vi "File_Application Path Keeper.vi"(6 "Skip Dialogue":bool, 8 "Error":errorcluster, 11 "File Keeper Files":T1) -> (0 "Error Out":errorcluster, 2 "Valid Item Out":bool, 3 "Path Out":path=path "D:/Pitney PTS/PTS PROGRAMS/2-Sparks 1 and 2/SparksMain32.vi")   [LabVIEW 2015]
uses:
  TypeDefs_Utility/ENUM_File Keeper List.ctl
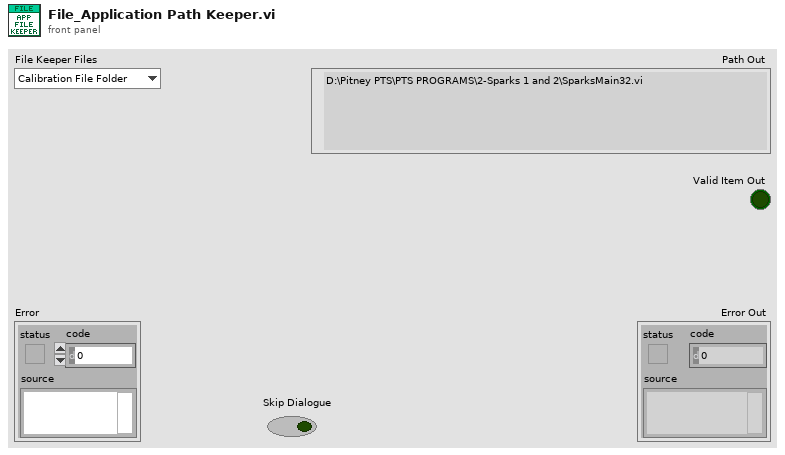
[diagram p1: front panel]
types:
  T1 = typedef "ENUM_File Keeper List.ctl" = enum16{"Calibration File Folder", "PNG Image Folder", "CSV File Folder"}
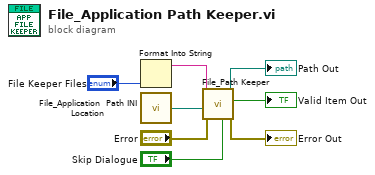
[diagram p0: block diagram]
diagram:
  n1 = Format Into String("File Keeper Files") -> (resulting string=w6:string)  [unwired: 3 in, 1 out]
  n2 = call "File_Application  Path INI Location.vi"() -> ("Path INI Location"=w8:path)
  n3 = call "File_Path Keeper.vi"("Skip Dialogue"="Skip Dialogue", "Error"="Error", "INI File Path"=w8, "File / Directory Name"=w6) -> ("Error Out"=→"Error Out":errorcluster, "Valid Item Out"=→"Valid Item Out":bool, "Path Out"=→"Path Out":path)  [unwired: 5 in]
